vi "Read Elements.vi"(8 "error in (no error)":errorcluster, 11 "Structure in":refnum<class "Structure.lvclass">) -> (0 "error out":errorcluster, 2 "Elements":refnum<class "Geometric.lvclass">[](array[class]), 3 "Structure out":refnum<class "Structure.lvclass">)   [LabVIEW 2019, in "Structure.lvclass"]
uses:
  Structure.lvclass
  Structure.lvclass/Structure.ctl
  Elements/Geometric.lvclass
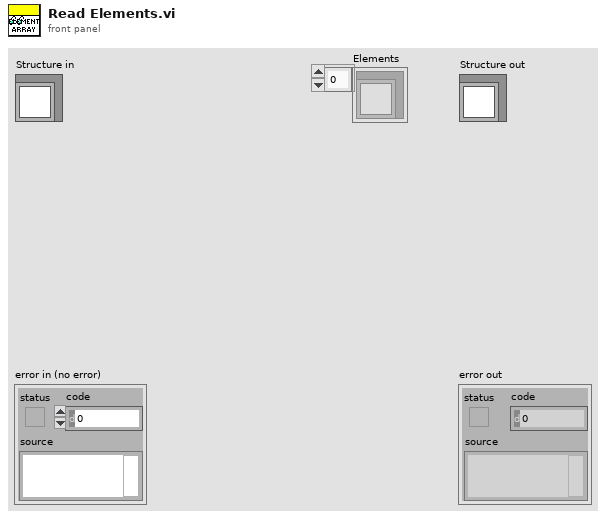
[diagram p1: front panel]
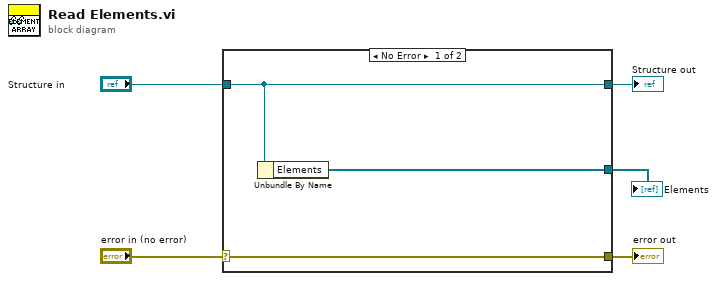
[diagram p0: block diagram]
diagram:
  n1 = case shown="No Error" "error in (no error)" {
    selector: "error in (no error)" -> [w8 w9]
    tunnel: [w8 w9] -> w4
    tunnel: [w7 w10] -> w2
    tunnel: "Structure in" -> [w7 w10]
    tunnel: [w6 _] -> w1
    frame No Error {
      n2 = Unbundle By Name(w7) -> ("Elements"=w6:refnum<class "Geometric.lvclass">[])
    }
    frame Error {
    }
  }
  "error out" <- w4
  "Structure out" <- w2
  "Elements" <- w1
